vi "memory to strings.vi"(8 "error in":errorcluster, 11 "memory hierarchy":T4) -> (0 "error out":errorcluster, 3 "1.0.0":T1)   [LabVIEW 2013, in "NISE_CEF_TreeSerializer.lvlib"]
uses:
  NISE_CEF_TreeSerializer.lvlib
  memory hierarchy.ctl
  hierarchy element.ctl
  serializable configuration/NISE_CEF_serializable configuration.lvclass
  file data format.ctl
  instance data.ctl
  serializable configuration/NISE_CEF_serializable configuration.lvclass/NISE_CEF_serializable configuration.ctl
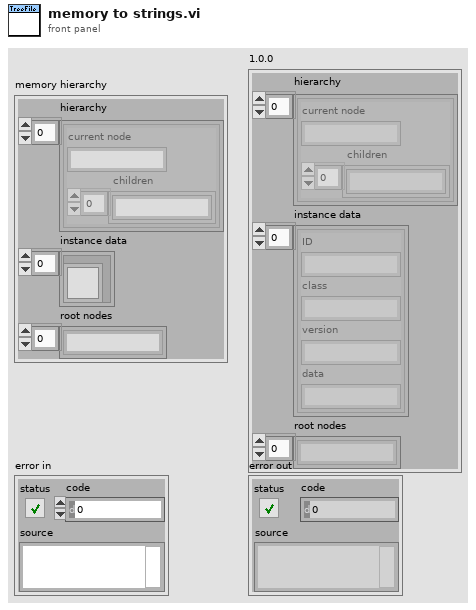
[diagram p1: front panel]
types:
  T1 = typedef "NISE_CEF_TreeSerializer.lvlib/file data format.ctl" = cluster{"hierarchy":T2[], "instance data":T3[], "root nodes":string[]}
  T2 = typedef "NISE_CEF_TreeSerializer.lvlib/hierarchy element.ctl" = cluster{"current node":string, "children":string[]}
  T3 = typedef "NISE_CEF_TreeSerializer.lvlib/instance data.ctl" = cluster{"ID":string, "class":string, "version":string, "data":string}
  T4 = typedef "NISE_CEF_TreeSerializer.lvlib/memory hierarchy.ctl" = cluster{"hierarchy":T2[], "instance data":refnum<class "NISE_CEF_serializable configuration.lvclass">[], "root nodes":string[]}
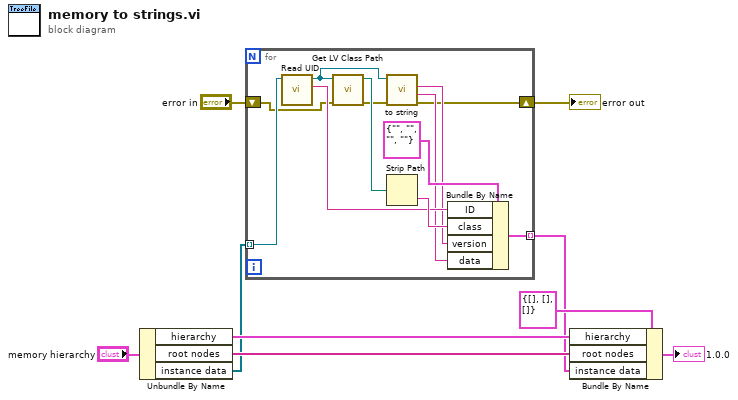
[diagram p0: block diagram]
diagram:
  n1 = Unbundle By Name("memory hierarchy") -> ("hierarchy"=w6:T2[], "root nodes"=w5:string[], "instance data"=w3:refnum<class "NISE_CEF_serializable configuration.lvclass">[])
  n2 = for {
    tunnel: [w20] -> w4 mode=indexing
    tunnel: w3 -> [w17] mode=indexing
    shift-right: [w11] -> w2
    shift-left: "error in" -> [w10]
    n3 = call "Read UID.vi"("configuration in"=w17) -> ("instance id"=w16:string, "configuration out"=w13:refnum<class "NISE_CEF_serializable configuration.lvclass">)  [unwired: 8 in, 1 out]
    n4 = call <vilib>:"Get LV Class Path.vi"("error in (no error)"=w10, "object"=w13) -> ("error out"=w12:errorcluster, "class path"=w19:path)  [unwired: 8 in]
    n5 = call-dynamic "to string.vi"("error in"=w12, "configuration in"=w13) -> ("error out"=w11:errorcluster, "data"=w14:string, "version"=w15:string)  [unwired: 6 in, 1 out]
    n6 = Strip Path(path=w19) -> (name=w18:string)  [unwired: 1 out]
    n7 = Bundle By Name(cluster=T3 {"ID"="", "class"="", "version"="", "data"=""} ("instancedata"), "ID"=w16, "class"=w18, "version"=w15, "data"=w14) -> (w20:T3)
  }
  "error out" <- w2
  n8 = Bundle By Name(cluster=T1 {"hierarchy"=[], "instance data"=[], "root nodes"=[]} ("1.0.0"), "hierarchy"=w6, "root nodes"=w5, "instance data"=w4) -> (→"1.0.0":T1)
